vi "Generate Waveform.vi"(8 "error in (no error)":errorcluster) -> (0 "error out":errorcluster, 3 "Data":dbl[](graph))   [LabVIEW 2025, in "Scope.lvlib" / "Sim Scope.lvclass"]
uses:
  Sim Scope.lvclass
  <vilib>/ptbypt/NI_PtbyPt.lvlib
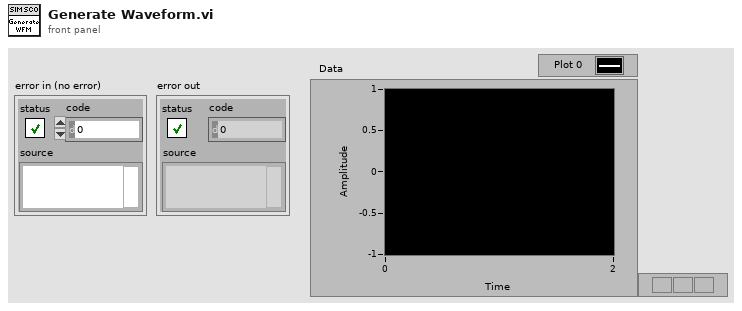
[diagram p1: front panel]
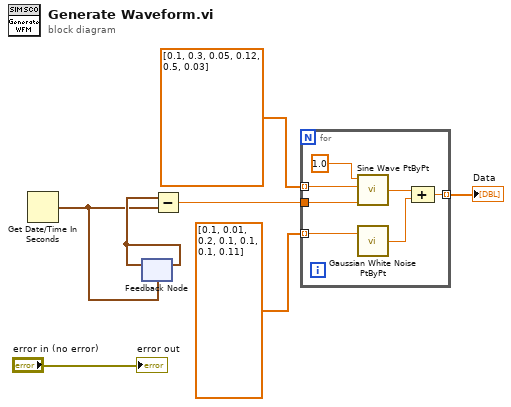
[diagram p0: block diagram]
diagram:
  n1 = Get Date/Time In Seconds() -> (seconds since 1Jan1904=w5:timestamp)
  n2 = feedback #1(w5) -> (w7:timestamp)
  n3 = feedback-in #1(w7) -> ()
  n4 = Subtract(x=w7, y=w5) -> (x-y=w6:dbl)
  n5 = for {
    tunnel: w6 -> [w12]
    tunnel: [w11] -> w2 mode=indexing
    tunnel: dbl[] [0.1, 0.3, 0.05, 0.12, 0.5, 0.03] ("frequency") -> [w9] mode=indexing
    tunnel: dbl[] [0.1, 0.01, 0.2, 0.1, 0.1, 0.1, 0.11] ("standard deviation") -> [w8] mode=indexing
    n6 = call <vilib>:"Sine Wave PtByPt.vi"("time"=w12, "frequency"=w9, "amplitude"=1.0) -> ("sine wave"=w14:dbl)  [unwired: 1 in]
    n7 = call <vilib>:"Gaussian White Noise PtByPt.vi"("standard deviation"=w8) -> ("Gaussian white noise"=w13:dbl)  [unwired: 2 in]
    n8 = Compound Arithmetic op=ADD(w14, w13) -> (w11:dbl)
  }
  "Data" <- w2
  "error out" <- "error in (no error)"
